vi "Prepend Parent Information.vi"(10 "Prepend String":string, 11 "Control Information in":string[][](array[string])) -> (3 "Control Information out":string[][](array[string]))   [LabVIEW 2017, in "Localization.lvlib"]
doc: "From the Control Information, takes the first column and adds 7 spaces, the Prepend String and a \"::\" in front of the nested control name so it is clear it is part of the cluster, table or other composite control.\n\nChoose Movement Consulting, LLC"
uses:
  Localization.lvlib
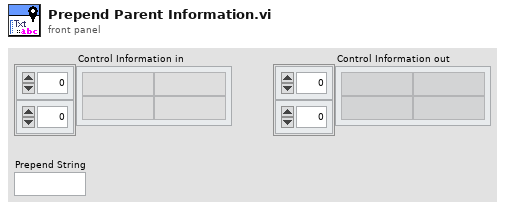
[diagram p1: front panel]
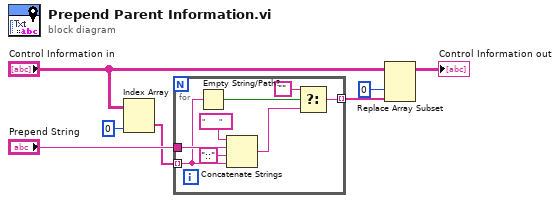
[diagram p0: block diagram]
diagram:
  n1 = Index Array(array="Control Information in", index (col)=0 ("disabled index (col)")) -> (element=w2:string[])  [unwired: 1 in]
  n2 = for {
    tunnel: w2 -> [w12] mode=indexing
    tunnel: "Prepend String" -> [w15]
    tunnel: [w8] -> w7 mode=indexing
    n3 = Empty String/Path?(string/path=w12) -> (empty?=w11:bool)
    n4 = Concatenate Strings("       " ("string"), w15, "::" ("string"), w12) -> (w9:string)
    n5 = Select(t="", s=w11, f=w9) -> (s? t:f=w8:string)
  }
  n6 = Replace Array Subset(array="Control Information in", new element=w7, index (col)=0 ("disabled index (col)")) -> (→"Control Information out":string[][])  [unwired: 1 in]
